vi "quickDisplayVariant.vi"() -> ()   [LabVIEW 2020]
panel:
  out "data":variant
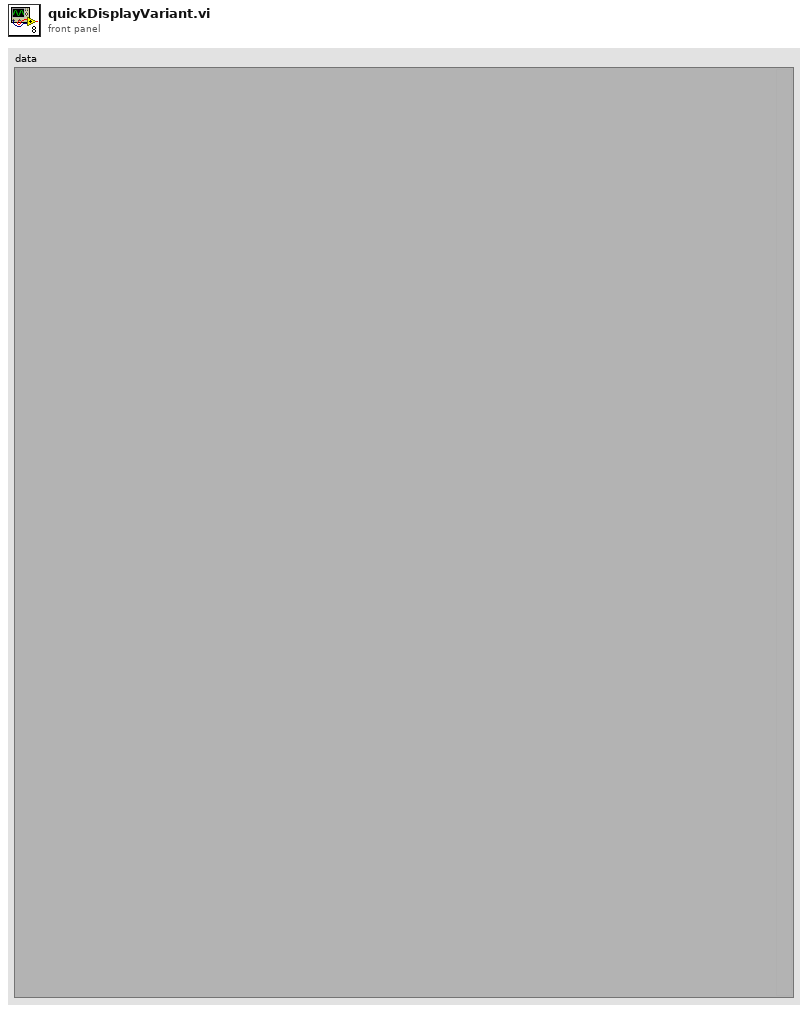
[diagram p1: front panel]
types:
  T1 = enum16{"Read", "Write", "ReadWrite", "BufferedRead", "BufferedReadWrite"}
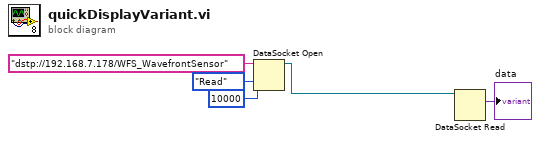
[diagram p0: block diagram]
diagram:
  n1 = DataSocket Open(9:10000 ("ms timeout (10000)"), 10:T1."Read" ("mode"), 11:"dstp://192.168.7.178/WFS_WavefrontSensor" ("URL")) -> (3:w2:refnum<k13>)  [unwired: 1 in, 1 out]
  n2 = DataSocket Read(11:w2) -> (2:→"data":variant)  [unwired: 4 in, 6 out]
